vi "PositionFromOrigin.vi"(11 "Position Info":T1) -> ()   [LabVIEW 2017]
uses:
  TypeDefs/Position-Info-TD.ctl
  Globals/Trav-Positon-Info.vi
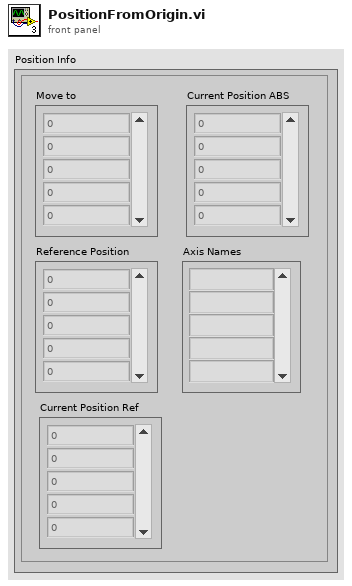
[diagram p1: front panel]
types:
  T1 = typedef "Position-Info-TD.ctl" = cluster{"Current Position ABS":dbl[], "Move to":dbl[], "Reference Position":dbl[], "Axis Names":string[], "Current Position Ref":dbl[]}
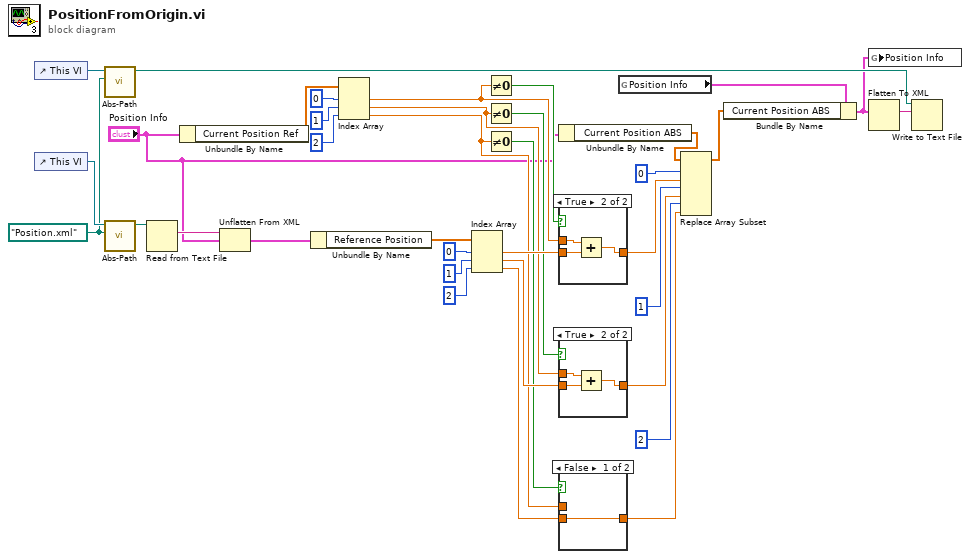
[diagram p0: block diagram]
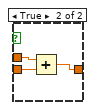
[diagram p2: hidden frame]
diagram:
  w13 = path "Position.xml" ("file (use dialog)")
  n1 = control-ref of="This VI"() -> (w17:refnum<vi>)
  n2 = control-ref of="This VI"() -> (w32:refnum<vi>)
  n3 = call "Abs-Path.vi"("filename"=w13, "Vi in path"=w17) -> ("Full path"=w18:path)  [unwired: 9 in]
  n4 = call "Abs-Path.vi"("filename"=w13, "Vi in path"=w32) -> ("Full path"=w31:path)  [unwired: 9 in]
  n5 = Read from Text File(file (use dialog)=w31) -> (text=w33:string)  [unwired: 3 in, 3 out]
  n6 = Unbundle By Name("Position Info") -> ("Current Position Ref"=w6:dbl[])
  n7 = Unflatten From XML(xml string=w33, type="Position Info") -> (value=w12:T1)  [unwired: 1 in, 1 out]
  n8 = Unbundle By Name(w12) -> ("Reference Position"=w10:dbl[])
  n9 = Index Array(array=w6, index #1=0 ("index"), index #2=1 ("index"), index #3=2 ("index")) -> (element #1=w5:dbl, element #2=w4:dbl, element #3=w3:dbl)
  n10 = Index Array(array=w10, index #1=0 ("index"), index #2=1 ("index"), index #3=2 ("index")) -> (element #1=w23:dbl, element #2=w25:dbl, element #3=w24:dbl)
  n11 = Not Equal To 0?(x=w5) -> (x != 0?=w27:bool)
  n12 = Not Equal To 0?(x=w4) -> (x != 0?=w19:bool)
  n13 = Not Equal To 0?(x=w3) -> (x != 0?=w20:bool)
  n14 = Unbundle By Name("Position Info") -> ("Current Position ABS"=w2:dbl[])
  n15 = case shown="True" w27 {
    tunnel: w5 -> [_ w40]
    tunnel: [w37 w39] -> w26
    tunnel: w23 -> [w37 w38]
    frame False {
    }
    frame True {
      n16 = Add(x=w40, y=w38) -> (x+y=w39:dbl)
    }
  }
  n17 = case shown="True" w19 {
    tunnel: w4 -> [_ w44]
    tunnel: [w41 w43] -> w21
    tunnel: w25 -> [w41 w42]
    frame False {
    }
    frame True {
      n18 = Add(x=w44, y=w42) -> (x+y=w43:dbl)
    }
  }
  n19 = case shown="False" w20 {
    tunnel: w3 -> [_ w48]
    tunnel: [w45 w47] -> w22
    tunnel: w24 -> [w45 w46]
    frame False {
    }
    frame True {
      n20 = Add(x=w48, y=w46) -> (x+y=w47:dbl)
    }
  }
  n21 = global read "Trav-Positon-Info.vi" "Position Info"() -> (w16:T1)
  n22 = Replace Array Subset(array=w2, new element #1=w26, index #1=0 ("index"), new element #2=w21, index #2=1 ("index"), new element #3=w22, index #3=2 ("index")) -> (w14:dbl[])
  n23 = Bundle By Name(cluster=w16, "Current Position ABS"=w14) -> (w15:T1)
  n24 = global write "Trav-Positon-Info.vi" "Position Info"(w15) -> ()
  n25 = Flatten To XML(anything=w15) -> (xml string=w11:string)
  n26 = Write to Text File(file (use dialog)=w18, text=w11) -> ()  [unwired: 2 in, 3 out]
